vi "Config Analog and Still Output.vi"(0 "VISA resource name":refnum<visa-resource-name>, 1 "Channel (1)":i32=1 min=1 max=16 step=1, 2 "High Value (0.00000E+0)":dbl min=0.0 max=100000000.0 step=1e-06 format="%^.5e", 3 "Low Value (0.00000E+0)":dbl min=0.0 max=100000000.0 step=1e-06 format="%^.5e", 5 "Analog Out Mode (0: Off)":u16(ring) items=["Off", "Channel", "Manual", "Zone", "Still"], 7 "Analog Channel (0: Analog Out 1)":u16(ring) items=["Analog Out 1", "Analog Out 2"], 9 "Source (0: Kelvin)":u16(ring) items=["Kelvin", "Ohms", "Linear Data"], 11 "error in (no error)":errorcluster, 12 "Bipolar Mode (F: OFF)":bool, 13 "Manual Value (0.000%)":dbl min=-100.0 max=100.0 step=0.001 format="%.3f", 14 "Still Value (0.000%)":dbl min=-100.0 max=100.0 step=0.001 format="%.3f") -> (4 "VISA resource name out":refnum<visa-resource-name>, 15 "error out":errorcluster)   [LabVIEW 2012, in "Lake Shore Cryotronics 370.lvlib"]
doc: "This VI configures the 370 analog outputs. The Model 370 has two analog voltage outputs designated ANALOG OUT 1 and ANALOG OUT 2 (STILL). They are variable DC voltage sources that can vary from +10V to -10V."
uses:
  <instrlib>/Lake Shore Cryotronics 370/Lake Shore Cryotronics 370.lvlib
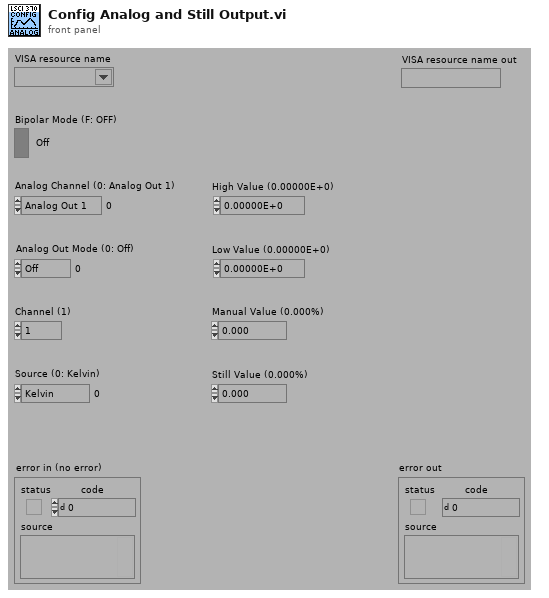
[diagram p1: front panel]
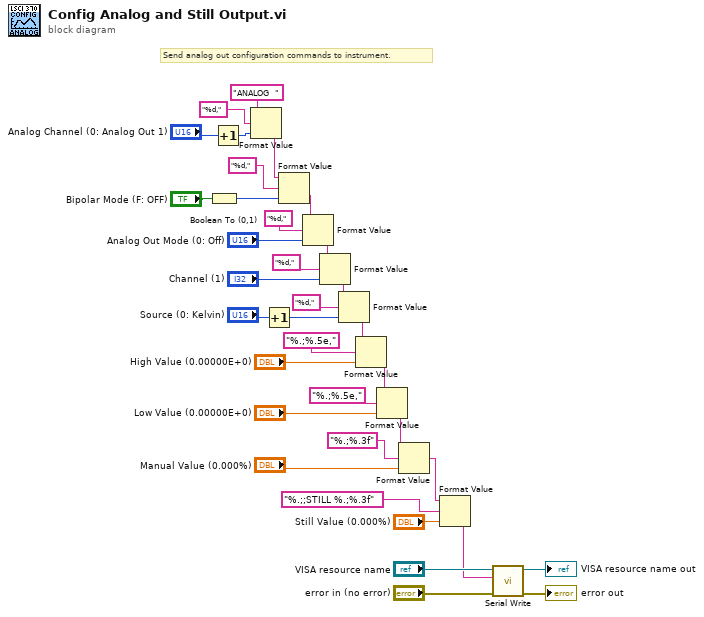
[diagram p0: block diagram]
diagram:
  # "Send analog out configuration commands to instrument."
  n1 = Boolean To (0,1)(Boolean="Bipolar Mode (F: OFF)") -> (0, 1=w29:i16)
  n2 = Increment(x="Analog Channel (0: Analog Out 1)") -> (x+1=w16:u16)
  n3 = Format Value(string ("")="ANALOG  ", format string="%d,", value (0)=w16) -> (output string=w14:string)
  n4 = Increment(x="Source (0: Kelvin)") -> (x+1=w24:u16)
  n5 = Format Value(string ("")=w14, format string="%d,", value (0)=w29) -> (output string=w27:string)
  n6 = Format Value(string ("")=w27, format string="%d,", value (0)="Analog Out Mode (0: Off)") -> (output string=w13:string)
  n7 = Format Value(string ("")=w13, format string="%d,", value (0)="Channel (1)") -> (output string=w12:string)
  n8 = Format Value(string ("")=w12, format string="%d,", value (0)=w24) -> (output string=w8:string)
  n9 = Format Value(string ("")=w8, format string="%.;%.5e,", value (0)="High Value (0.00000E+0)") -> (output string=w9:string)
  n10 = Format Value(string ("")=w9, format string="%.;%.5e,", value (0)="Low Value (0.00000E+0)") -> (output string=w7:string)
  n11 = Format Value(string ("")=w7, format string="%.;%.3f", value (0)="Manual Value (0.000%)") -> (output string=w3:string)
  n12 = Format Value(string ("")=w3, format string="%.;;STILL %.;%.3f", value (0)="Still Value (0.000%)") -> (output string=w1:string)
  n13 = call <instrlib>:"Serial Write.vi"("error in (no error)"="error in (no error)", "Write Buffer (\"\")"=w1, "VISA resource name"="VISA resource name") -> ("error out"=→"error out":errorcluster, "VISA resource name out"=→"VISA resource name out":refnum<visa-resource-name>)  [unwired: 6 in, 1 out]
